vi "Launch controls for file management.vi"(10 "date mod to Pass (hours) in":u8, 11 "File Management in":T1) -> (2 "date mod to Pass (hours) out":u8, 3 "File Management out":T1)   [LabVIEW 2011]
doc: "Will launch a vi to set file management methods"
uses:
  Controls/File Management.ctl
panel:
  in  "set file extentions":bool
  in  "Cancel Button":bool
  in  "OK Button":bool
  in  "time date mod":bool
  # "Set Your File Handle Methods"
  # "File Handling Method"
  # "File Handling Method"
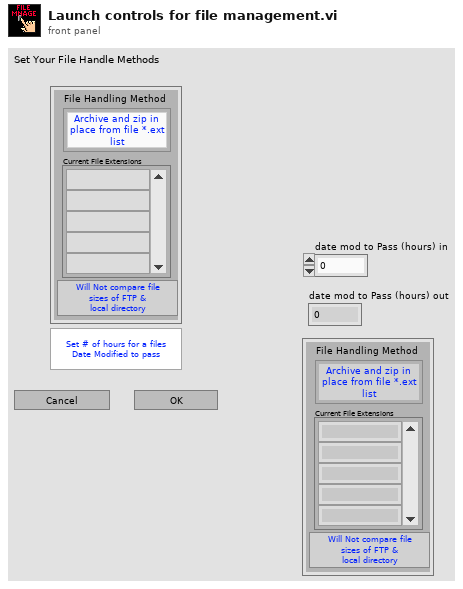
[diagram p1: front panel]
types:
  T1 = typedef "File Management.ctl" = cluster{"Comp File Size":bool, "File Handle Method":enum16{"Archive and zip in place from file *.ext list", "Archive and zip ALL file Types to archive directory", "Archive and zip to archive directory from file *.ext list", "Perform no file management"}, "file extention list":string[]}
  T2 = enum16{"Archive and zip in place from file *.ext list", "Archive and zip ALL file Types to archive directory", "Archive and zip to archive directory from file *.ext list", "Perform no file management"}
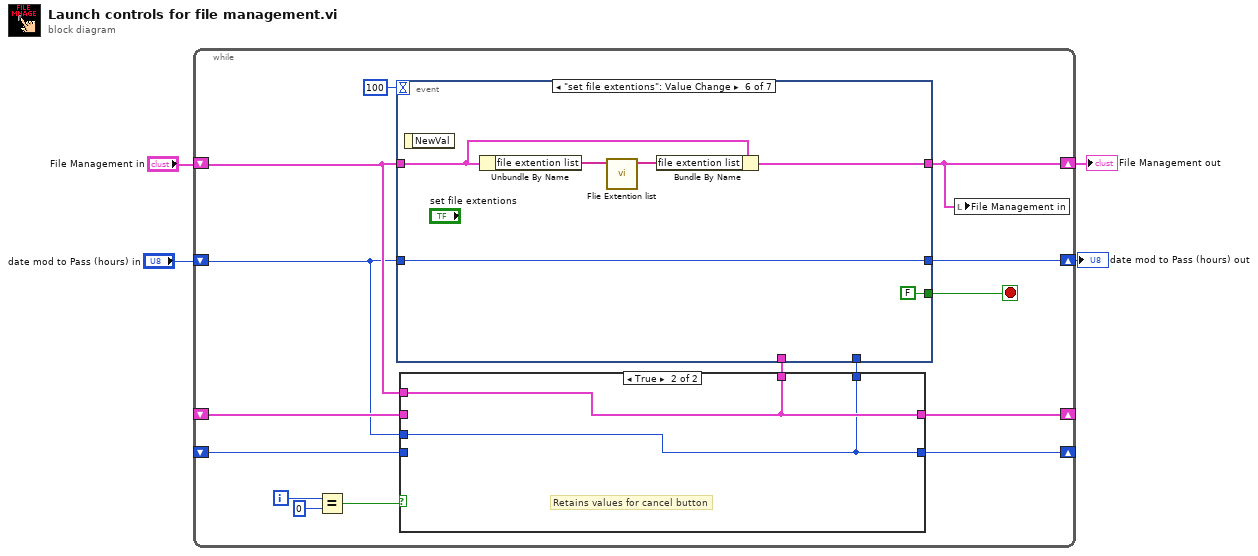
[diagram p0: block diagram]
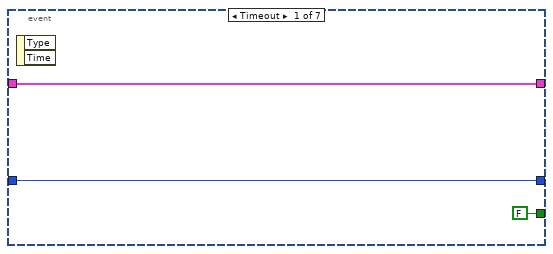
[diagram p3: hidden frame]
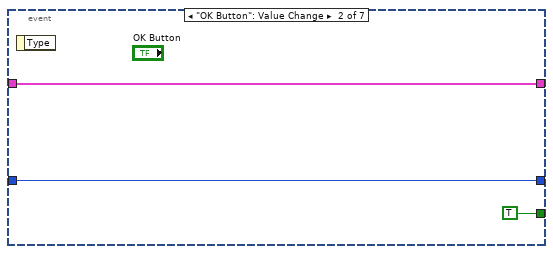
[diagram p4: hidden frame]
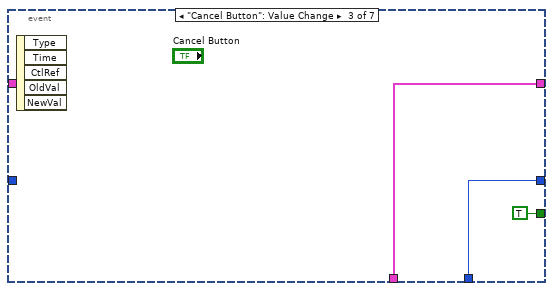
[diagram p5: hidden frame]
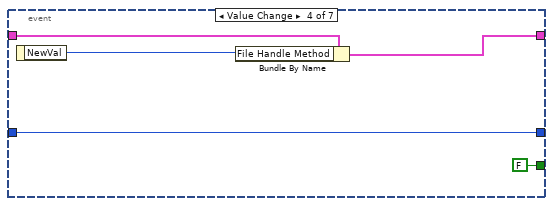
[diagram p6: hidden frame]
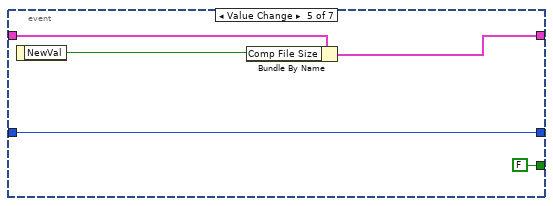
[diagram p7: hidden frame]
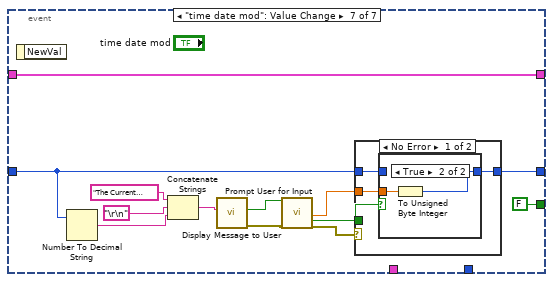
[diagram p8: hidden frame]
diagram:
  n1 = while {
    shift-right: [w14] -> _
    shift-left: _ -> [w12]
    shift-right: [w11] -> _
    shift-left: _ -> [w10]
    shift-right: [w5] -> w4
    shift-left: "File Management in" -> [w7]
    shift-right: [w13] -> w3
    shift-left: "date mod to Pass (hours) in" -> [w6]
    i -> [w17]
    stop <- w18 stop-if-true
    n2 = Equal?(x=w17, y=0) -> (x = y?=w15:bool)
    n3 = case shown="True" w15 {
      tunnel: w7 -> [_ w23]
      tunnel: [w21 w23] -> w14
      tunnel: w12 -> [w21 _]
      tunnel: w6 -> [_ w22]
      tunnel: [w20 w22] -> w11
      tunnel: w10 -> [w20 _]
      tunnel: [w21 w23] -> w9
      tunnel: [w20 w22] -> w8
      frame False {
      }
      frame True {
        # "Retains values for cancel button"
      }
    }
    n4 = event shown="[5] \"set file extentions\": Value Change" {
      selector: _ -> [_ _ _ _ _ _ _]
      dyn-events: _ -> [_ _ _ _ _ _ _]
      timeout: 100 -> [_ _ _ _ _ _ _]
      tunnel: [w26 w29 w32 w33 w38 w45 w51] -> w5
      tunnel: w7 -> [w26 w29 _ w35 w40 w44 w51]
      tunnel: w6 -> [w25 w28 _ w37 w42 w48 w52]
      tunnel: [w25 w28 w31 w37 w42 w48 w50] -> w13
      tunnel: [FALSE TRUE TRUE FALSE FALSE FALSE FALSE] -> w18
      tunnel: w9 -> [_ _ w32 _ _ _ _]
      tunnel: w8 -> [_ _ w31 _ _ _ _]
      event Timeout {
        n5 = event-data() -> ()  [unwired: 1 in, 2 out]
      }
      event "OK Button": Value Change {
        n6 = event-data() -> ()  [unwired: 1 in, 1 out]
      }
      event "Cancel Button": Value Change {
        n7 = event-data() -> ()  [unwired: 1 in, 5 out]
      }
      event Value Change {
        n8 = event-data() -> ("NewVal"=w34:T2)  [unwired: 1 in]
        n9 = Bundle By Name(cluster=w35, "File Handle Method"=w34) -> (w33:T1)
      }
      event Value Change {
        n10 = event-data() -> ("NewVal"=w39:bool)  [unwired: 1 in]
        n11 = Bundle By Name(cluster=w40, "Comp File Size"=w39) -> (w38:T1)
      }
      event "set file extentions": Value Change {
        n12 = event-data() -> ()  [unwired: 1 in, 1 out]
        n13 = Unbundle By Name(w44) -> ("file extention list"=w43:string[])
        n14 = call "Flie Extention list.vi"("file extention list IN"=w43) -> ("File extention list (out)"=w46:string[])  [unwired: 10 in]
        n15 = Bundle By Name(cluster=w44, "file extention list"=w46) -> (w45:T1)
      }
      event "time date mod": Value Change {
        n16 = event-data() -> ()  [unwired: 1 in, 1 out]
        n17 = Number To Decimal String(number=w52) -> (decimal integer string=w60:string)  [unwired: 1 in]
        n18 = Concatenate Strings("The Current number of hours that need to passed on a files last modified date before the file will be archived and moved to the ftp server." ("Message"), "\r\n", w60) -> (w58:string)
        n19 = call "Display Message to User"("Message"=w58) -> ("error out"=w55:errorcluster, "Change Value"=w56:bool)  [unwired: 9 in]
        n20 = call "Prompt User for Input"("Enable"=w56, "error in (no error)"=w55) -> ("(Hours)"=w54:dbl, "OK"=w53:bool, "error out"=w61:errorcluster)  [unwired: 15 in]
        n21 = case shown="No Error" w61 {
          tunnel: w53 -> [w65 _]
          tunnel: w54 -> [w64 _]
          tunnel: [w63 w69] -> w50
          tunnel: w52 -> [w62 w69]
          frame No Error {
            n22 = case shown="True" w65 {
              tunnel: w64 -> [_ w68]
              tunnel: w62 -> [w66 _]
              tunnel: [w66 w67] -> w63
              frame False {
              }
              frame True {
                n23 = To Unsigned Byte Integer(number=w68) -> (unsigned 8bit integer=w67:u8)
              }
            }
          }
          frame Error {
          }
        }
      }
    }
    n24 = local write "File Management in"(w5) -> ()
  }
  "date mod to Pass (hours) out" <- w3
  "File Management out" <- w4
